vi "H5D_read_1d_sgl.vi"(5 "name":string, 6 "error in (no error)":errorcluster, 9 "ref":i32) -> (0 "error out":errorcluster, 3 "ref out":i32, 4 "data":sgl[](array[numeric]))   [LabVIEW 2013]
uses:
  <vilib>/addons/h5labview/H5Base.lvlib
  <vilib>/addons/h5labview/hdf5dll.dll
  <vilib>/addons/h5labview/H5TypeSpace.lvlib
panel:
  in  "datatype":sgl
  # "h5labview :: H5D"
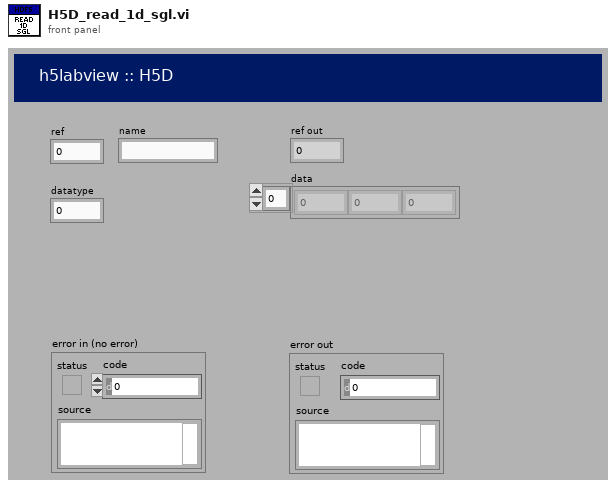
[diagram p1: front panel]
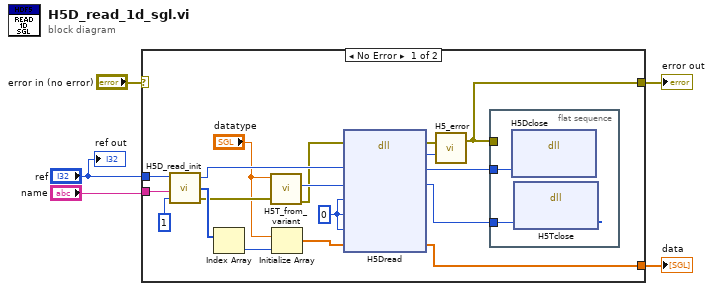
[diagram p0: block diagram]
diagram:
  n1 = case shown="No Error" "error in (no error)" {
    selector: "error in (no error)" -> [_ w26]
    tunnel: [w13 w26] -> w2
    tunnel: "ref" -> [w23 _]
    tunnel: "name" -> [w22 _]
    tunnel: [w12 _] -> w1
    frame No Error {
      w6 = 0 ("H5S_ALL")
      n2 = call <vilib>:"H5D_read_init.vi"("ndims"=1, "name"=w22, "ref"=w23) -> ("error out"=w14:errorcluster, "dims"=w16:u32[], "ds_id"=w17:i32)
      n3 = Index Array(array=w16) -> (element=w8:u32)  [unwired: 1 in]
      n4 = call <vilib>:"H5T_from_variant.vi"("error in (no error)"=w14, "type in"="datatype") -> ("error out"=w7:errorcluster, "h5type"=w11:i32)  [unwired: 2 in, 2 out]
      n5 = Initialize Array("datatype", w8) -> (w15:sgl[])
      n6 = dll-call lib="C:/Program Files (x86)/National Instruments/LabVIEW 2013/vi.lib/addons/h5labview/hdf5dll.dll" fn="H5Dread" label="hdf5_call"(error in=w7, "ds_id"=w17, "mem_type"=w11, "mem_space"=w6, "file_space_id"=w6, "xfer_plist_id"=w6, "buffer"=w15) -> (error out=w19:errorcluster, "return type"=w18:i32, "ds_id"=w21:i32, "mem_type"=w20:i32, "buffer"=w12:sgl[])  [unwired: 5 in, 1 out]
      n7 = call <vilib>:"H5_error.vi"("retval"=w18, "error in (no error)"=w19) -> ("error out"=w13:errorcluster)  [unwired: 1 in]
      n8 = flat-sequence {
        tunnel: w21 -> [w25]
        tunnel: w20 -> [w24]
        tunnel: w13 -> [_]
        frame #0 {
          n9 = dll-call lib="C:/Program Files (x86)/National Instruments/LabVIEW 2013/vi.lib/addons/h5labview/hdf5dll.dll" fn="H5Dclose" ("hdf5_call")("ds_id"=w25) -> ()  [unwired: 5 in, 2 out]
          n10 = dll-call lib="C:/Program Files (x86)/National Instruments/LabVIEW 2013/vi.lib/addons/h5labview/hdf5dll.dll" fn="H5Tclose" ("hdf5_call")("t_id"=w24) -> ()  [unwired: 5 in, 2 out]
        }
      }
    }
    frame Error {
    }
  }
  "error out" <- w2
  "data" <- w1
  "ref out" <- "ref"
